vi "libretrieve_request_parameter.vi"(8 "error in (no error)":errorcluster, 10 "id":string, 11 "output":i32) -> (0 "error out":errorcluster, 2 "parameter":string)   [LabVIEW 2015]
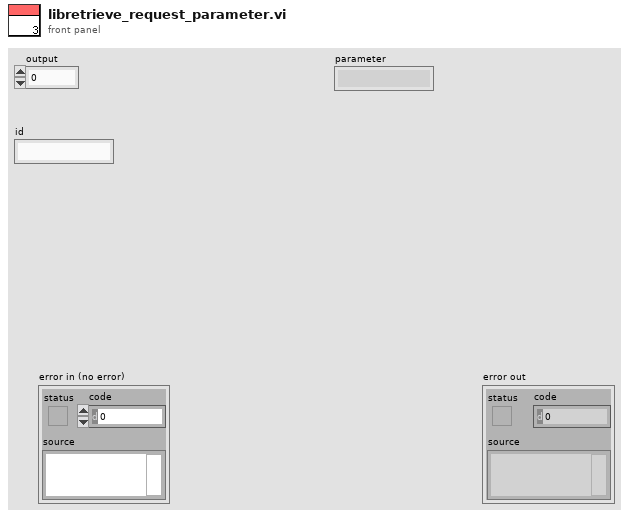
[diagram p1: front panel]
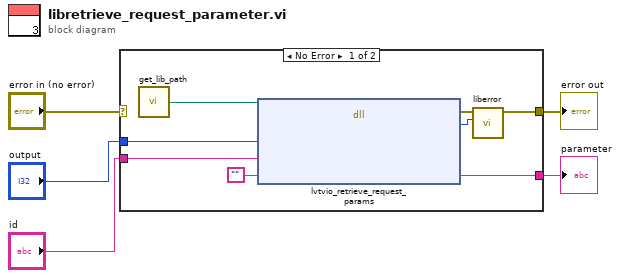
[diagram p0: block diagram]
diagram:
  n1 = case shown="No Error" "error in (no error)" {
    selector: "error in (no error)" -> [_ w14]
    tunnel: [w6 w14] -> w4
    tunnel: [w12 _] -> w2
    tunnel: "id" -> [w11 _]
    tunnel: "output" -> [w9 _]
    frame No Error {
      n2 = call "get_lib_path.vi"() -> ("Path"=w13:path)
      n3 = dll-call lib="S:/thingiverselv/lib/liblvtvio.dll" fn="lvtvio_retrieve_request_params"(path in=w13, "output"=w9, "id"=w11, "parameter"="") -> (error out=w8:errorcluster, "return type"=w7:i32, "parameter"=w12:string)  [unwired: 4 in, 1 out]
      n4 = call "liberror.vi"("tvio errors"=w7, "error in (no error)"=w8) -> ("error out"=w6:errorcluster)  [unwired: 9 in]
    }
    frame Error {
    }
  }
  "error out" <- w4
  "parameter" <- w2
